vi "Write Password.vi"(8 "error in (no error)":errorcluster, 11 "Master in":refnum<class "MASTER.lvclass">) -> (0 "error out":errorcluster, 3 "Master out":refnum<class "MASTER.lvclass">)   [LabVIEW 2014, in "Files Library.lvlib" / "Master.lvclass"]
uses:
  MASTER/MASTER.lvclass
  MASTER/MASTER.lvclass/MASTER.ctl
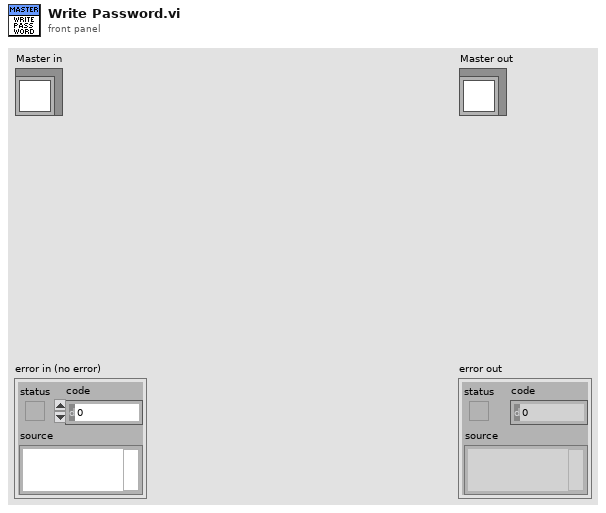
[diagram p1: front panel]
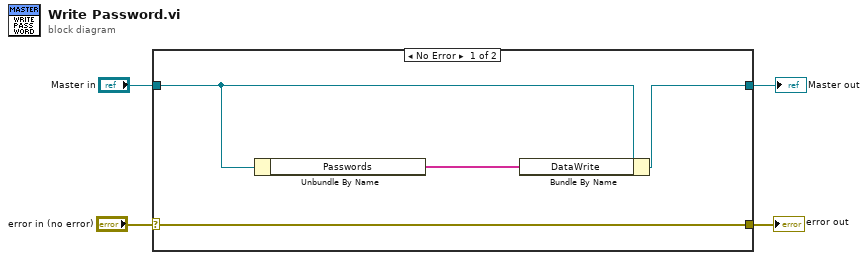
[diagram p0: block diagram]
diagram:
  n1 = case shown="No Error" "error in (no error)" {
    selector: "error in (no error)" -> [w8 w10]
    tunnel: [w8 w10] -> w3
    tunnel: [w7 w9] -> w1
    tunnel: "Master in" -> [w6 w9]
    frame No Error {
      n2 = Unbundle By Name(w6) -> ("Passwords"=w5:string[])
      n3 = Bundle By Name(cluster=w6, "DataWrite"=w5) -> (w7:refnum<class "MASTER.lvclass">)
    }
    frame Error {
    }
  }
  "error out" <- w3
  "Master out" <- w1
